vi "SWITCH Configure Auto Zero.vi"(8 "error in (no error)":errorcluster, 10 "Message Data":variant, 11 "Data Cluster in":T1={"Tango HW"={"VISA resource"="101:110", "Baud Rate (115200)"=0, "lAnInterfaceType"=0, "bAShowProt"=0}, "Writer Queue"=refnum, "Status"=FALSE, "Abs Position"=[], "Axis Velocity"={"dX"=0.0, "dY"=0.0, "dZ"=0.0, "dA"=0.0}, "acceleration "=0.0, "Z direction"=enum."Up", "Position Mode"="", "plLSID"=0}) -> (0 "error out":errorcluster, 3 "Data Cluster out":T1={"Tango HW"={"VISA resource"="101:110", "Baud Rate (115200)"=0, "lAnInterfaceType"=0, "bAShowProt"=0}, "Writer Queue"=refnum, "Status"=FALSE, "Abs Position"=[], "Axis Velocity"={"dX"=0.0, "dY"=0.0, "dZ"=0.0, "dA"=0.0}, "acceleration "=0.0, "Z direction"=enum."Up", "Position Mode"="", "plLSID"=0})   [LabVIEW 2020, in "MOTOR.lvlib"]
uses:
  MOTOR.lvlib
  support/Message Queue/Message Cluster.ctl
  support/Message Queue/Message Queue.lvlib
  PS Hardware Configuration.ctl
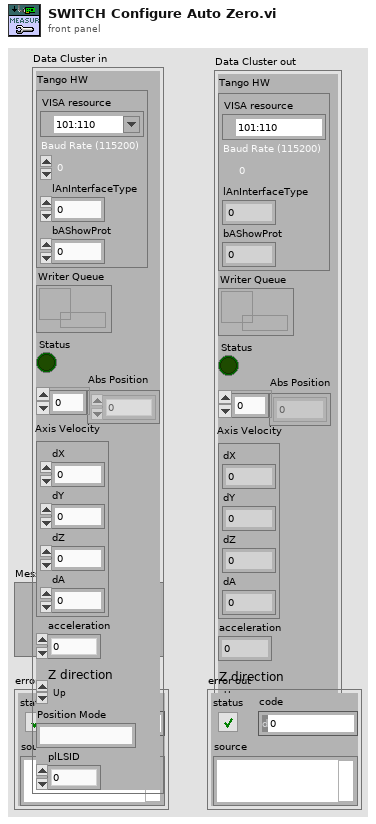
[diagram p1: front panel]
types:
  T1 = typedef "MOTOR.lvlib/PS Hardware Configuration.ctl" = cluster{"Tango HW":cluster{"VISA resource":refnum<visa-resource-name>, "Baud Rate (115200)":i32, "lAnInterfaceType":i32, "bAShowProt":i32}, "Writer Queue":refnum<queue>, "Status":bool, "Abs Position":i32[], "Axis Velocity":cluster{"dX":dbl, "dY":dbl, "dZ":dbl, "dA":dbl}, "acceleration ":dbl, "Z direction":enum16{"Up", "Down"}, "Position Mode":string, "plLSID":i32}
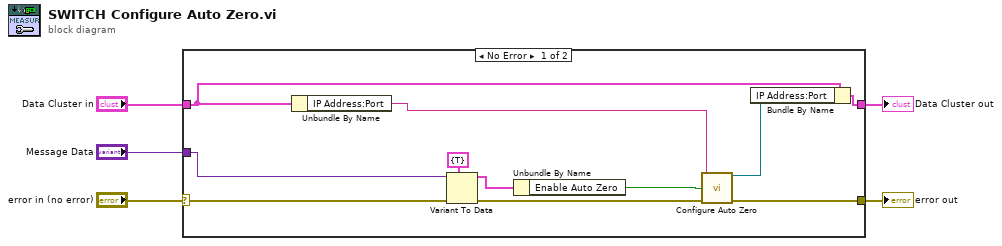
[diagram p0: block diagram]
diagram:
  n1 = case shown="No Error" "error in (no error)" {
    selector: "error in (no error)" -> [w7 w17]
    tunnel: "Message Data" -> [w8 _]
    tunnel: [w16 w18] -> w4
    tunnel: "Data Cluster in" -> [w15 w18]
    tunnel: [w11 w17] -> w2
    frame No Error {
      n2 = Unbundle By Name(w15) -> ("IP Address:Port"=w13:string)
      n3 = Variant To Data(error in=w7, type=cluster{"Enable Auto Zero":bool} {"Enable Auto Zero"=TRUE}, Variant=w8) -> (data=w14:cluster{"Enable Auto Zero":bool}, error out=w10:errorcluster)
      n4 = Unbundle By Name(w14) -> ("Enable Auto Zero"=w6:bool)
      n5 = call <instrlib>:"Configure Auto Zero.vi"("VISA resource name"=w13, "Enable Auto Zero (True)"=w6, "error in (no error)"=w10) -> ("VISA resource name out"=w12:refnum<visa-resource-name>, "error out"=w11:errorcluster)  [unwired: 11 in]
      n6 = Bundle By Name(cluster=w15, "IP Address:Port"=w12) -> (w16:T1)
    }
    frame Error {
    }
  }
  "Data Cluster out" <- w4
  "error out" <- w2
